vi "Snake Template.vi"(11 "Data In":T3={"Time Limit"=1000, "Length"=0, "Memory"=[], "Barrier"=[[-1, -1, -1], [-1, -255, -1], [-1, -1, -1]], "Snake"=[[-1, -1, -1], [-1, -255, -1], [-1, -1, -1]], "Tail"=[[-1, -1, -1], [-1, -255, -1], [-1, -1, -1]], "Food"=[[-1, -1, -1], [-1, -255, -1], [-1, -1, -1]]}) -> (3 "Data Out":T1)   [LabVIEW 2015]
doc: "Created IvanLis by LabVIEW Portal\nProfile: http://labviewportal.org/memberlist.php?mode=viewprofile&u=987\neMail: IvanLisanov@gMail.com"
uses:
  Snake TypeDef/Snake DataIn TypeDef.ctl
  Snake TypeDef/Snake DataOut TypeDef.ctl
  TypeDef/Direction_TypeDef.ctl
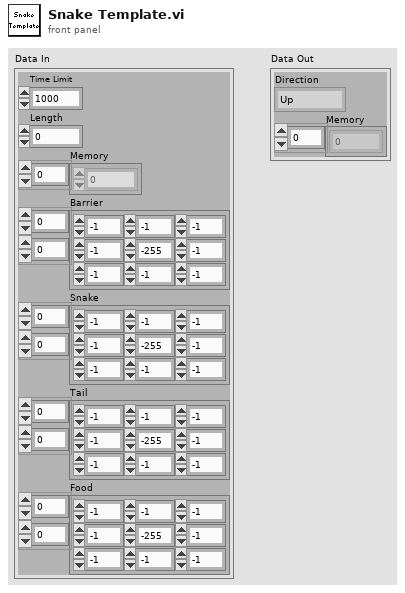
[diagram p1: front panel]
types:
  T1 = typedef "Snake DataOut TypeDef.ctl" = cluster{"Direction":T2, "Memory":u8[]}
  T2 = typedef "Direction_TypeDef.ctl" = enum8{"Up", "Down", "Left", "Right"}
  T3 = typedef "Snake DataIn TypeDef.ctl" = cluster{"Time Limit":i32, "Length":i32, "Memory":u8[], "Barrier":i32[][], "Snake":i32[][], "Tail":i32[][], "Food":i32[][]}
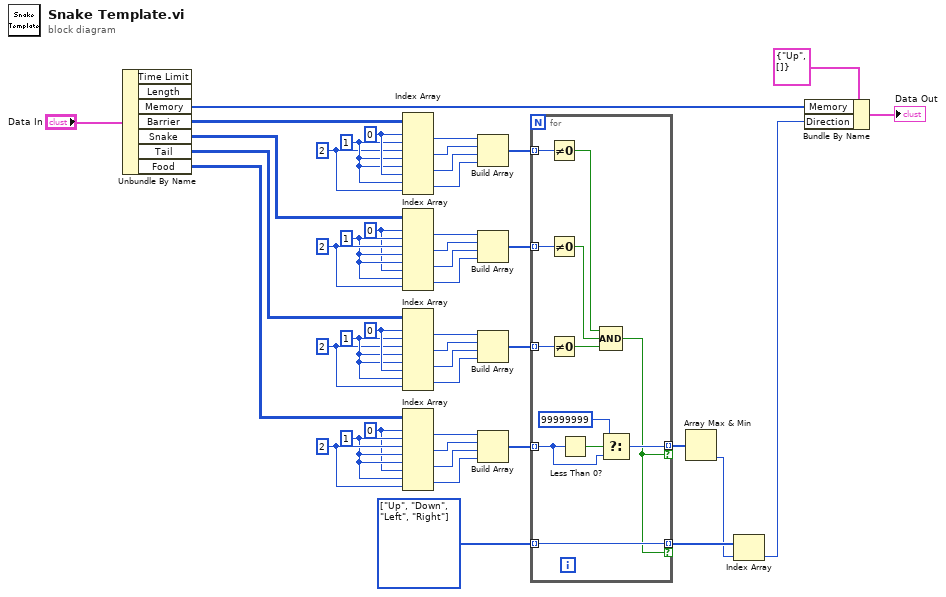
[diagram p0: block diagram]
diagram:
  w16 = 2 ("index (row)")
  w15 = 1 ("disabled index (col)")
  w14 = 0 ("index (row)")
  w25 = 2 ("index (row)")
  w26 = 1 ("disabled index (col)")
  w27 = 0 ("index (row)")
  w30 = 2 ("index (row)")
  w29 = 1 ("disabled index (col)")
  w28 = 0 ("index (row)")
  w39 = 2 ("index (row)")
  w6 = T2[] [enum."Up", enum."Down", enum."Left", enum."Right"] items=["Up", "Down", "Left", "Right"] ("Array")
  w40 = 1 ("disabled index (col)")
  w41 = 0 ("index (row)")
  n1 = Unbundle By Name("Data In") -> ("Memory"=w1:u8[], "Barrier"=w42:i32[][], "Snake"=w13:i32[][], "Tail"=w12:i32[][], "Food"=w11:i32[][])  [unwired: 2 out]
  n2 = Index Array(array=w42, index (row) #1=w41, index (col) #1=w40, index (row) #2=w39, index (col) #2=w40, index (row) #3=w40, index (col) #3=w41, index (row) #4=w40, index (col) #4=w39) -> (element #1=w38:i32, element #2=w37:i32, element #3=w36:i32, element #4=w35:i32)
  n3 = Index Array(array=w13, index (row) #1=w28, index (col) #1=w29, index (row) #2=w30, index (col) #2=w29, index (row) #3=w29, index (col) #3=w28, index (row) #4=w29, index (col) #4=w30) -> (element #1=w31:i32, element #2=w32:i32, element #3=w33:i32, element #4=w34:i32)
  n4 = Index Array(array=w12, index (row) #1=w27, index (col) #1=w26, index (row) #2=w25, index (col) #2=w26, index (row) #3=w26, index (col) #3=w27, index (row) #4=w26, index (col) #4=w25) -> (element #1=w24:i32, element #2=w23:i32, element #3=w22:i32, element #4=w21:i32)
  n5 = Index Array(array=w11, index (row) #1=w14, index (col) #1=w15, index (row) #2=w16, index (col) #2=w15, index (row) #3=w15, index (col) #3=w14, index (row) #4=w15, index (col) #4=w16) -> (element #1=w17:i32, element #2=w18:i32, element #3=w19:i32, element #4=w20:i32)
  n6 = Build Array(w38, w37, w36, w35) -> (w10:i32[])
  n7 = Build Array(w31, w32, w33, w34) -> (w9:i32[])
  n8 = Build Array(w24, w23, w22, w21) -> (w8:i32[])
  n9 = Build Array(w17, w18, w19, w20) -> (w7:i32[])
  n10 = for {
    tunnel: w10 -> [w54] mode=indexing
    tunnel: w9 -> [w53] mode=indexing
    tunnel: w8 -> [w52] mode=indexing
    tunnel: w7 -> [w50] mode=indexing
    tunnel: w6 -> [w47] mode=indexing
    tunnel: [w48] -> w5 mode=indexing if=w46
    tunnel: [w47] -> w4 mode=indexing if=w46
    n11 = Not Equal To 0?(x=w54) -> (x != 0?=w57:bool)
    n12 = Not Equal To 0?(x=w53) -> (x != 0?=w56:bool)
    n13 = Not Equal To 0?(x=w52) -> (x != 0?=w55:bool)
    n14 = Less Than 0?(x=w50) -> (x < 0?=w51:bool)
    n15 = Compound Arithmetic op=AND(w57, w56, w55) -> (w46:bool)
    n16 = Select(t=99999999, s=w51, f=w50) -> (s? t:f=w48:i32)
  }
  n17 = Array Max & Min(array=w5) -> (min index (indices)=w3:i32)  [unwired: 3 out]
  n18 = Index Array(array=w4, index=w3) -> (element=w2:T2)
  n19 = Bundle By Name(cluster=T1 {"Direction"=enum."Up", "Memory"=[]} ("Data Out"), "Memory"=w1, "Direction"=w2) -> (→"Data Out":T1)
